vi "Do.vi"(8 "error in (no error)":errorcluster, 10 "Actor in":refnum<class "Actor.lvclass">, 11 "Data Update Msg":refnum<class "Data Update Msg.lvclass">) -> (0 "error out":errorcluster, 2 "Actor out":refnum<class "Actor.lvclass">)   [LabVIEW 2011, in "Data Update Msg.lvclass"]
doc: "(<B>Filename</B>: Actor Framework.lvlib:Message.lvclass:Do.vi)\n\nDefines what a message does when it is received by an actor. Generally, a message instructs an actor to invoke one of its methods.\n\nBy default, this method does nothing. A child class must override it to define behavior. Create a child class by using the Actor Framework Message Maker dialog box."
uses:
  Data Update Msg.lvclass
  <userlib>/_Frameworks/ActorFramework/Actor/Actor.lvclass
  Actors/Controller/Controller.lvclass
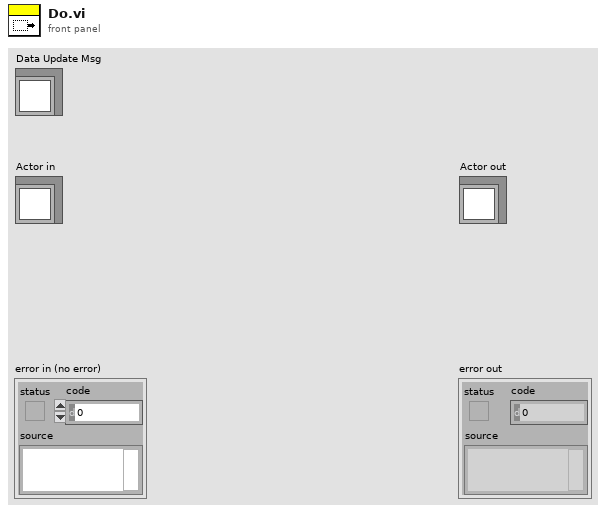
[diagram p1: front panel]
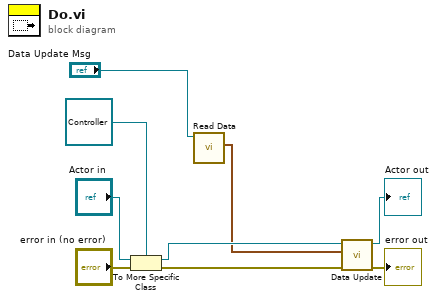
[diagram p0: block diagram]
diagram:
  n1 = To More Specific Class(target class=refnum<class "Controller.lvclass"> refnum ("Controller.lvclass"), reference="Actor in", error in="error in (no error)") -> (specific class reference=w3:refnum<class "Controller.lvclass">, error out=w8:errorcluster)
  n2 = call "Read Data.vi"("Data Update Msg in"="Data Update Msg") -> ("Data"=w1:cluster{"EDR":dbl, "Pulse":u8})  [unwired: 9 in, 1 out]
  n3 = call-dynamic "Data Update.vi"("error in (no error)"=w8, "Data"=w1, "Controller in"=w3) -> ("error out"=→"error out":errorcluster, "Controller out"=→"Actor out":refnum<class "Controller.lvclass">)  [unwired: 7 in]
